vi "LV86_Save JPG.vi"(2 "Path to file":path, 3 "Image":T1 {"Dialogs" format="%.0b"}) -> (1 "Image":T1 {"Dialogs" format="%.0b"})   [LabVIEW 2024]
doc: "This VI saves an image to a JPEG file."
uses:
  <userlib>/ImageProcessing/QTLIB_2595_LV86/QT_Private.ctl
  <userlib>/ImageProcessing/QTLIB_2595_LV86/QT_File.ctl
  <userlib>/ImageProcessing/QTLIB_2595_LV86/QT_Compression.ctl
  <userlib>/ImageProcessing/QTLIB_2595_LV86/QT_Image.ctl
panel:
  in  "Format":u16(ring)=1 items=["BMP", "JPEG", "MacPaint", "Photoshop", "PNG", "PICT", "QuickTime", "SG", "Targa", "TIFF"]
  in  "Compression":i32(slide)=1023 scale=0.0..1023.0 scale format="%.0x"
  out "error out":errorcluster
  out "Path":path
  # "This VI saves an image to a JPEG file."
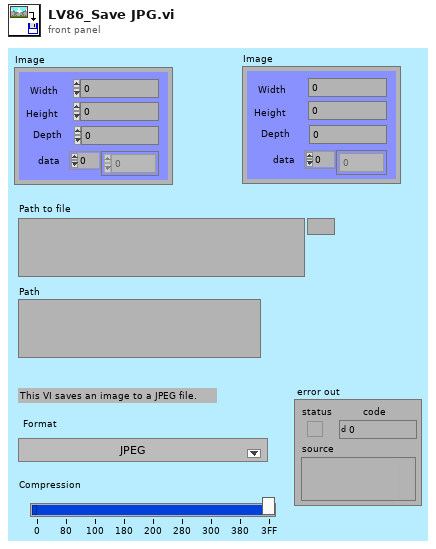
[diagram p1: front panel]
types:
  T1 = typedef "QT_Image.ctl" = cluster{"Width":i32, "Height":i32, "Depth":i32, "data":u8[], "Compressed data":u8[], "Color table":u32[], "Duration":i32, "Options":i32, "Timestamp":i32, "ID":i32, "Reserved":i32, "Dialogs":u32}
  T2 = typedef "QT_Compression.ctl" = cluster{"Compression":i32, "Format":i32, "Codec":i32, "Comp. Quality":i32, "Key Frame":i32, "Dialogs":u32}
  T3 = typedef "QT_File.ctl" = cluster{"Paths":string[], "Options":i32, "Dialogs":u32, "Reserved":i32}
  T4 = typedef "QT_Private.ctl" = cluster{"reserved 1":i32, "reserved 2":i32, "reserved 3":i32, "reserved 4":i32}
  T5 = typedef "imagedata.ctl" = cluster{"image type":i32, "image depth":i32, "image":u8[], "mask":u8[], "colors":u32[], "Rectangle":cluster{"left":i16, "top":i16, "right":i16, "bottom":i16}}
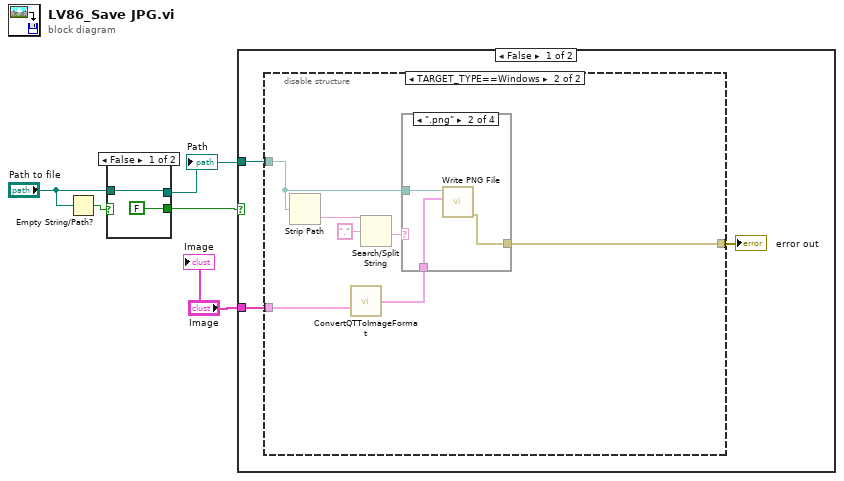
[diagram p0: block diagram]
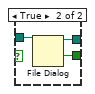
[diagram p2: hidden frame]
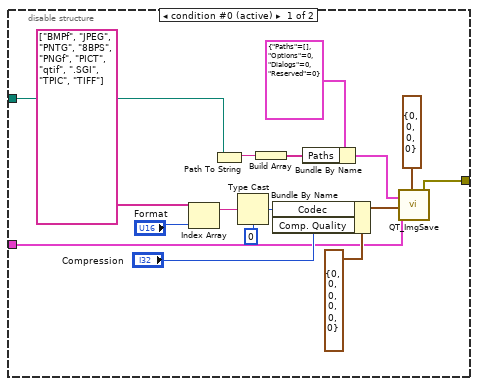
[diagram p3: hidden frame]
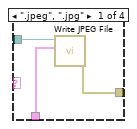
[diagram p4: hidden frame]
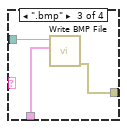
[diagram p5: hidden frame]
diagram:
  n1 = Empty String/Path?(string/path="Path to file") -> (empty?=w1:bool)
  n2 = case shown="False" w1 {
    tunnel: [FALSE ("cancelled") w10] -> w5
    tunnel: [w7 w9] -> w4
    tunnel: "Path to file" -> [w7 w8]
    frame False {
    }
    frame True {
      n3 = File Dialog(11:w8) -> (1:w10:bool, 3:w9:path)  [unwired: 1 in, 7 out]
    }
  }
  "Path" <- w4
  n4 = case shown="False" w5 {
    tunnel: w4 -> [w12 _]
    tunnel: "Image" -> [w11 _]
    frame False {
      n5 = disable-structure shown="TARGET_TYPE==Windows" {
        disable-tunnel: [w20 w30] -> w13
        disable-tunnel: w12 -> [w15 w33]
        disable-tunnel: w11 -> [w14 w32]
        frame condition #0 (active) {
          n6 = Index Array(array=string[] ["BMPf", "JPEG", "PNTG", "8BPS", "PNGf", "PICT", "qtif", ".SGI", "TPIC", "TIFF"], index="Format") -> (element=w26:string)
          n7 = Path To String(path=w15) -> (string=w16:string)
          n8 = Type Cast(type=0 ("Format"), x=w26) -> (*(type *) &x=w28:i32)
          n9 = Build Array(w16) -> (w29:string[])
          n10 = Bundle By Name(cluster=T2 {"Compression"=0, "Format"=0, "Codec"=0, "Comp. Quality"=0, "Key Frame"=0, "Dialogs"=0} ("Compression Settings"), "Codec"=w28, "Comp. Quality"="Compression") -> (w18:T2)
          n11 = Bundle By Name(cluster=T3 {"Paths"=[], "Options"=0, "Dialogs"=0, "Reserved"=0} ("File Settings"), "Paths"=w29) -> (w21:T3)
          n12 = call <userlib>:"QT_ImgSave.vi"("File Settings"=w21, "Image In"=w14, "Compression Settings"=w18, "Private"=T4 {"reserved 1"=0, "reserved 2"=0, "reserved 3"=0, "reserved 4"=0}) -> ("error out"=w20:errorcluster)  [unwired: 5 in, 10 out]
        }
        frame condition #1 {
          n13 = Strip Path(path=w33) -> (name=w36:string)  [unwired: 1 out]
          n14 = call <vilib>:"ConvertQTToImageFormat.vi"("Image In"=w32) -> ("image data out"=w31:T5)
          n15 = Search/Split String(string=w36, search string/char (-)=".") -> (match + rest of string=w34:string)  [unwired: 1 in, 2 out]
          n16 = case shown="\".png\"" w34 {
            tunnel: w33 -> [w39 w42 w45 _]
            tunnel: [w38 w41 w44 _] -> w30
            tunnel: w31 -> [w37 w40 w43 _]
            frame ".jpeg", ".jpg" {
              n17 = call <vilib>:"Write JPEG File.vi"("image data"=w37, "path to JPEG file"=w39) -> ("error out"=w38:errorcluster)  [unwired: 8 in, 1 out]
            }
            frame ".png" {
              n18 = call <vilib>:"Write PNG File.vi"("image data"=w40, "path to PNG file"=w42) -> ("error out"=w41:errorcluster)  [unwired: 8 in, 1 out]
            }
            frame ".bmp" {
              n19 = call <vilib>:"Write BMP File.vi"("image data"=w43, "path to BMP file"=w45) -> ("error out"=w44:errorcluster)  [unwired: 8 in, 1 out]
            }
            frame Default {
            }
          }
        }
      }
      "error out" <- w13
    }
    frame True {
    }
  }
  "Image" <- "Image"
